vi "img test14(coutsegment attempt1).vi"() -> ()   [LabVIEW 2013]
uses:
  <vilib>/vision/NI_Vision_Development_Module.lvlib
panel:
  out "Waveform Chart":i32(graph)
  in  "ON":bool
  out "s? t:f 2":i32[](array[numeric])
  out "s? t:f":i32[](array[numeric])
  out "Top player court segment display":bool[][](array[boolean])
  out "Bottom player court segment display":bool[][](array[boolean])
  out "bottom player":cluster{"Numeric":dbl, "Numeric":dbl}[](array[cluster])
  out "top player":cluster{"Numeric":dbl, "Numeric":dbl}[](array[cluster])
  in  "playing":bool
  out "Top VIew":cluster{"Numeric":dbl, "Numeric":dbl}[](graph)
  out "Image 4":T1(plugin-control)
  in  "frame jump":i32=3
  in  "speed":u32(slide)=200
  in  "start":i32(slide) step=219843704 scale=0.0..42095.0
  out "Image 3":T1(plugin-control)
  in  "AVI Path":path=path "C:/Users/Kokum Weeratunga/Desktop/img processing/ChenJin vs HuYun.avi"
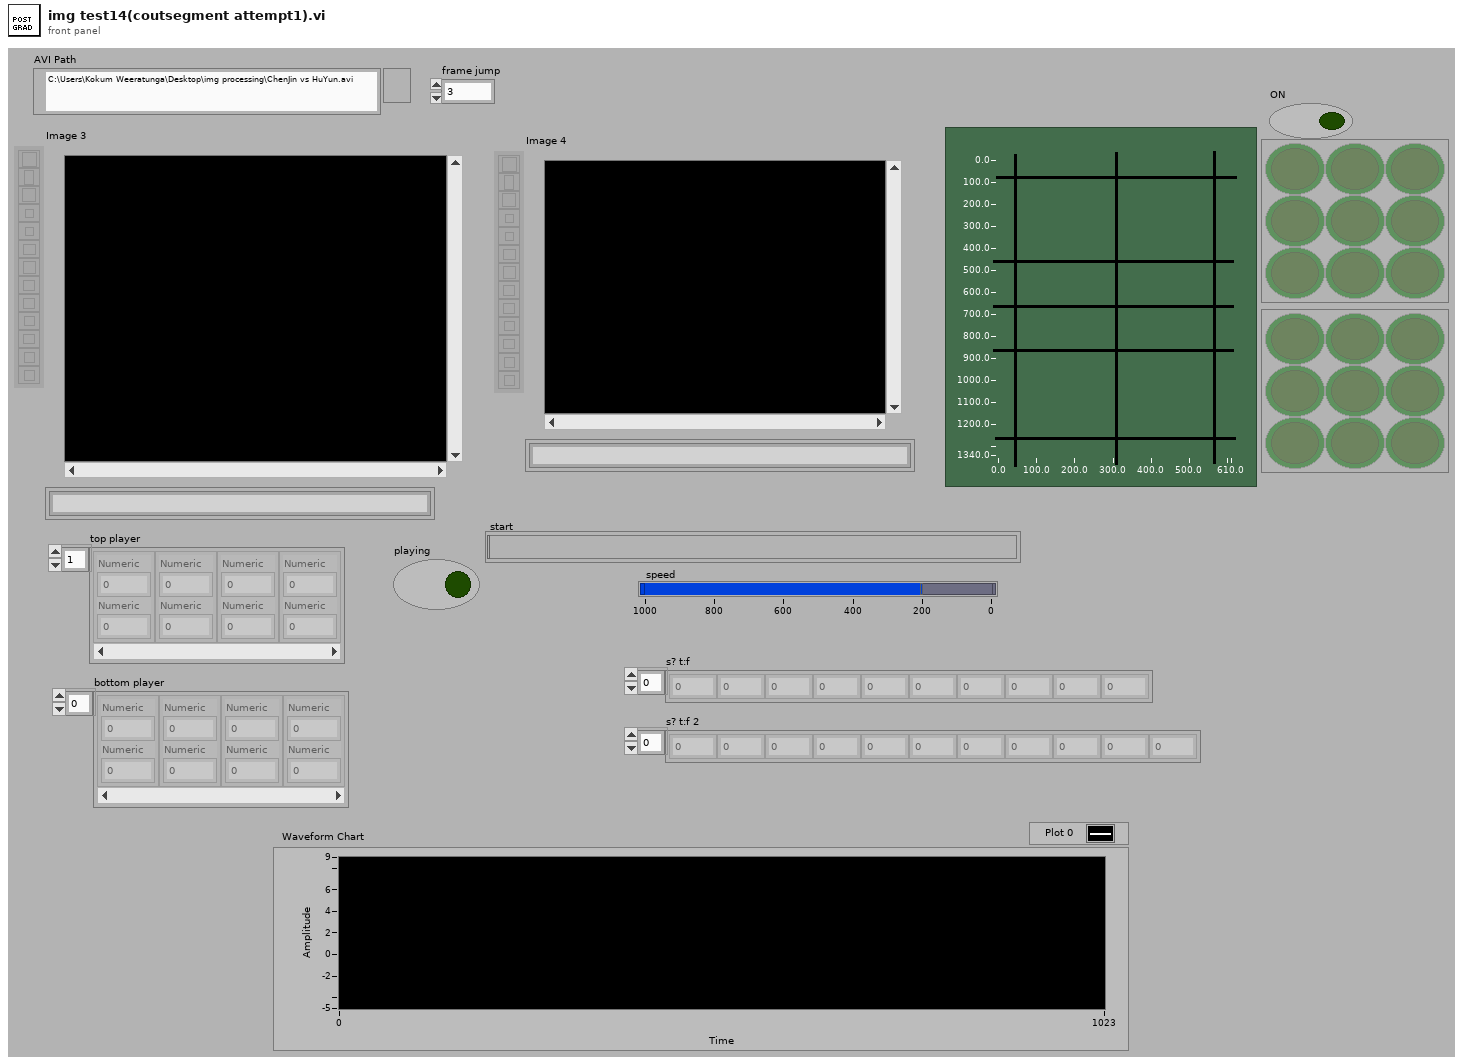
[diagram p1: front panel]
types:
  T1 = typedef "IMAQ Image.ctl" = refnum<image>
  T2 = typedef "Image Type" = u32
  T3 = typedef "AviRefnum.ctl" = refnum<k1>
  T4 = cluster{"width":u32, "height":u32, "framesPerSecond":u32, "compressionFilter":string, "hasData":bool}
  T5 = cluster{cluster{"X":sgl, "Y":sgl}[], cluster{i32, i32}[], "Unit":u32}
  T6 = cluster{"Origin Pixel":cluster{"X":sgl, "Y":sgl}, "Angle Relative to Horizontal (deg)":sgl, "Axis Reference":u32}
  T7 = typedef "Particle Parameters" = i32
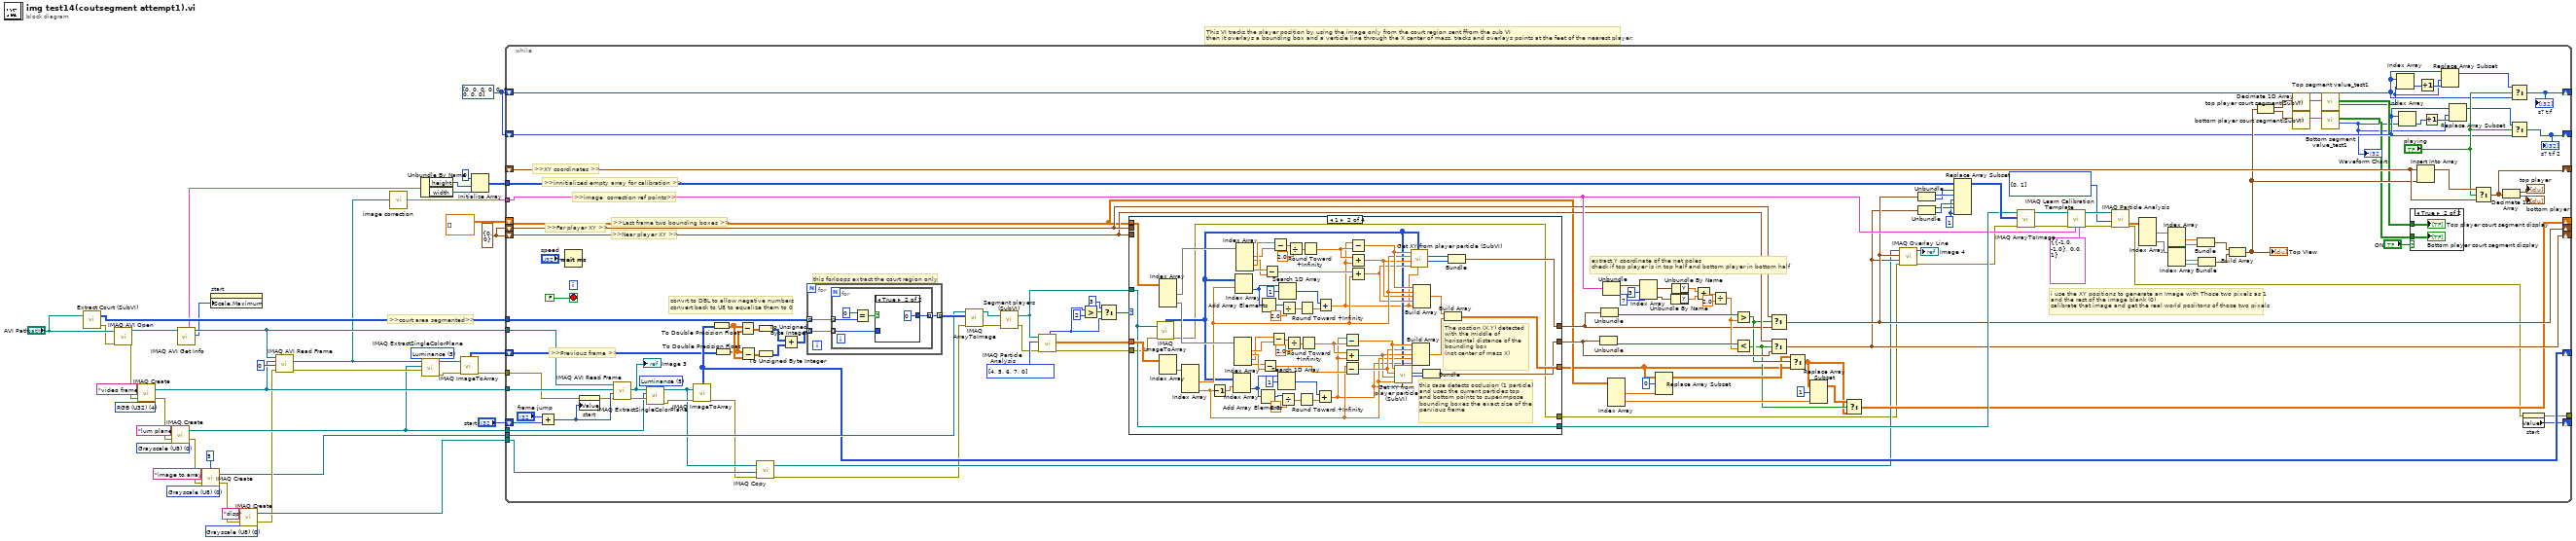
[diagram p0: block diagram]
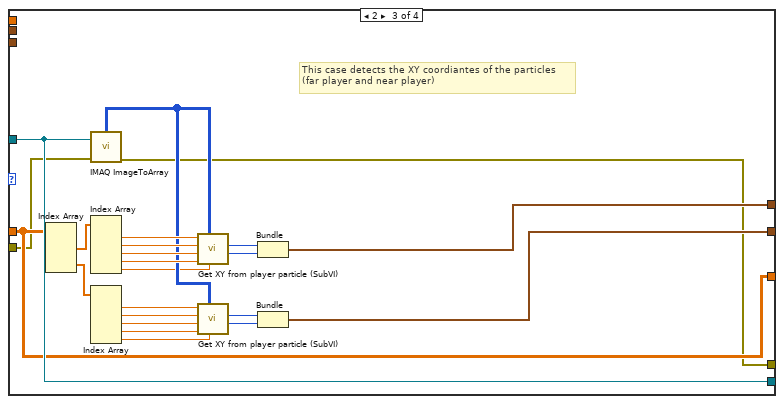
[diagram p4: hidden frame]
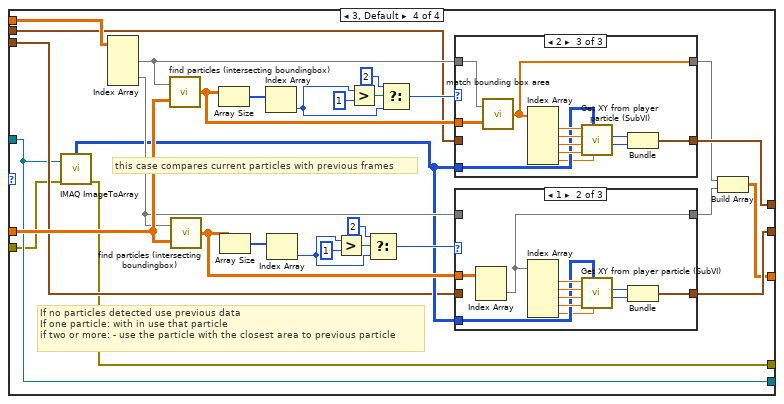
[diagram p5: hidden frame]
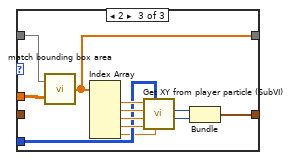
[diagram p7: hidden frame]
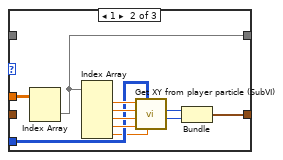
[diagram p9: hidden frame]
diagram:
  w1 = i32[] [0, 0, 0, 0, 0, 0, 0, 0, 0] ("input array")
  w14 = cluster{"X coordinate":i32, "Y coordinate":i32} {"X coordinate"=0, "Y coordinate"=0}
  w27 = T2 0 items=["Grayscale (U8)", "Grayscale (I16)", "Grayscale (SGL)", "Complex (CSG)", "RGB (U32)", "HSL (U32)", "RGB (U64)", "Grayscale (U16)"] ("Image Type")
  w34 = 5 items=["Red", "Green", "Blue", "Hue", "Saturation", "Luminance", "Value", "Intensity"] ("Color Plane")
  w35 = T2 0 items=["Grayscale (U8)", "Grayscale (I16)", "Grayscale (SGL)", "Complex (CSG)", "RGB (U32)", "HSL (U32)", "RGB (U64)", "Grayscale (U16)"] ("Image Type")
  w39 = T2 0 items=["Grayscale (U8)", "Grayscale (I16)", "Grayscale (SGL)", "Complex (CSG)", "RGB (U32)", "HSL (U32)", "RGB (U64)", "Grayscale (U16)"] ("Image Type")
  w37 = T2 4 items=["Grayscale (U8)", "Grayscale (I16)", "Grayscale (SGL)", "Complex (CSG)", "RGB (U32)", "HSL (U32)", "RGB (U64)", "Grayscale (U16)"] ("Image Type")
  # ">>court area segmented>>"
  # "This VI tracks the player position by using the image only from the court region sent ffrom the sub VI\nthen it overlays a bounding box and a verticle line through the X center of mass. tracks and overlays points at the feet of the nearest player."
  n1 = call "Extract Court (SubVI).vi"("AVI Path"="AVI Path") -> ("error out"=w41:errorcluster, "Court pixels out"=w17:u8[][])  [unwired: 1 in]
  n2 = call "IMAQ AVI Open"("error in (no error)"=w41, "AVI Path"="AVI Path") -> ("error out"=w23:errorcluster, "Avi Refnum"=w12:T3)  [unwired: 8 in]
  n3 = call "IMAQ Create"("Image Name"="video frame", "Image Type"=w37, "error in (no error)"=w23) -> ("New Image"=w31:T1, "error out"=w22:errorcluster)  [unwired: 2 in]
  n4 = call "IMAQ Create"("Image Name"="lum plane", "Image Type"=w39, "error in (no error)"=w22) -> ("New Image"=w30:T1, "error out"=w21:errorcluster)  [unwired: 2 in]
  n5 = call "IMAQ AVI Get Info"("Avi Refnum"=w12) -> ("Number of Frames"=w10:u32, "Avi Refnum (duplicate)"=w11:T3, "Frame Data"=w7:T4)  [unwired: 6 in, 2 out]
  n6 = call "IMAQ Create"("Border Size"=5, "Image Name"="image to array", "Image Type"=w35, "error in (no error)"=w21) -> ("New Image"=w16:T1, "error out"=w20:errorcluster)  [unwired: 1 in]
  n7 = property on="start" class="Slide (strict)"("Scale.Maximum"=w10) -> ()  [unwired: 2 in, 2 out]
  n8 = call "IMAQ Create"("Image Name"="disp", "Image Type"=w27, "error in (no error)"=w20) -> ("New Image"=w25:T1, "error out"=w19:errorcluster)  [unwired: 2 in]
  n9 = call "IMAQ AVI Read Frame"("error in (no error)"=w19, "Frame Number"=u32 0, "Image"=w31, "Avi Refnum"=w11) -> ("error out"=w33:errorcluster, "Image Out"=w3:T1)  [unwired: 4 in, 2 out]
  n10 = call "image correction.vi"("Image"=w3) -> ("ref points"=w2:T5)
  n11 = Unbundle By Name(w7) -> ("height"=w6:u32, "width"=w5:u32)
  n12 = call "IMAQ ExtractSingleColorPlane"("Color Plane"=w34, "error in (no error)"=w33, "Image Dst"=w30, "Image Src"=w3) -> ("error out"=w24:errorcluster, "Image Dst Out"=w28:T1)  [unwired: 6 in]
  n13 = call "IMAQ ImageToArray"("error in (no error)"=w24, "Image"=w28) -> ("error out"=w9:errorcluster, "Image Pixels (U8)"=w29:u8[][])  [unwired: 2 in, 3 out]
  n14 = Initialize Array(u8 0 ("element"), w6, w5) -> (w4:u8[][])
  n15 = while {
    tunnel: w11 -> [w134]
    tunnel: w31 -> [w153]
    tunnel: w17 -> [w169]
    tunnel: w30 -> [w154]
    tunnel: w16 -> [w166]
    shift-right: [w165] -> _
    shift-left: w29 -> [w164]
    tunnel: w25 -> [w137]
    shift-right: [w72] -> _
    shift-left: dbl[][] [] ("Particle Measurements (Pixels)") -> [w82]
    shift-right: [w86] -> _
    shift-left: w14 -> [w88]
    shift-right: [w84] -> _
    shift-left: w14 -> [w87]
    shift-right: [w130] -> _
    shift-left: "start" -> [w136]
    tunnel: w9 -> [w132]
    tunnel: w4 -> [w129]
    tunnel: w2 -> [w101]
    shift-right: [w104] -> _
    shift-left: _ -> [w107]
    shift-right: [w61] -> _
    shift-left: w1 -> [w52]
    shift-right: [w60] -> _
    shift-left: w1 -> [w56]
    tunnel: [w50] -> _
    stop <- FALSE stop-if-true
    w116 = T7[] [0, 1] items=["Center of Mass X", "Center of Mass Y", "First Pixel X", "First Pixel Y", "Bounding Rect Left", "Bounding Rect Top", "Bounding Rect Right", "Bounding Rect Bottom", "Max Feret Diameter Start X", "Max Feret Diameter Start Y", "Max Feret Diameter End X", "Max Feret Diameter End Y", "Max Horiz. Segment Length Left", "Max Horiz. Segment Length Right", "Max Horiz. Segment Length Row", "-", "Bounding Rect Width", "Bounding Rect Height", "Bounding Rect Diagonal", "Perimeter", "Convex Hull Perimeter", "Holes' Perimeter", "Max Feret Diameter", "Equivalent Ellipse Major Axis", "Equivalent Ellipse Minor Axis", "Equivalent Ellipse Minor Axis (Feret)", "Equivalent Rect Long Side", "Equivalent Rect Short Side", "Equivalent Rect Diagonal", "Equivalent Rect Short Side (Feret)", "Average Horiz. Segment Length", "Average Vert. Segment Length", "Hydraulic Radius", "Waddel Disk Diameter", "-", "Area", "Holes' Area", "Particle & Holes' Area", "Convex Hull Area", "Image Area", "-", "Number of Holes", "Number of Horiz. Segments", "Number of Vert. Segments", "-", "Orientation", "Max Feret Diameter Orientation", "-", "% Area/Image Area", "% Area/(Particle & Holes' Area)", "Ratio of Equivalent Ellipse Axes", "Ratio of Equivalent Rect Sides", "-", "Elongation Factor", "Compactness Factor", "Heywood Circularity Factor", "Type Factor", "-", "Sum X", "Sum Y", "Sum XX", "Sum XY", "Sum YY", "Sum XXX", "Sum XXY", "Sum XYY", "Sum YYY", "-", "Moment of Inertia XX", "Moment of Inertia XY", "Moment of Inertia YY", "Moment of Inertia XXX", "Moment of Inertia XXY", "Moment of Inertia XYY", "Moment of Inertia YYY", "Norm. Moment of Inertia XX", "Norm. Moment of Inertia XY", "Norm. Moment of Inertia YY", "Norm. Moment of Inertia XXX", "Norm. Moment of Inertia XXY", "Norm. Moment of Inertia XYY", "Norm. Moment of Inertia YYY", "Hu Moment 1", "Hu Moment 2", "Hu Moment 3", "Hu Moment 4", "Hu Moment 5", "Hu Moment 6", "Hu Moment 7"] ("Real-World Measurements")
    w124 = u8 1 ("new element/subarray")
    w155 = T7[] [4, 5, 6, 7, 0] items=["Center of Mass X", "Center of Mass Y", "First Pixel X", "First Pixel Y", "Bounding Rect Left", "Bounding Rect Top", "Bounding Rect Right", "Bounding Rect Bottom", "Max Feret Diameter Start X", "Max Feret Diameter Start Y", "Max Feret Diameter End X", "Max Feret Diameter End Y", "Max Horiz. Segment Length Left", "Max Horiz. Segment Length Right", "Max Horiz. Segment Length Row", "-", "Bounding Rect Width", "Bounding Rect Height", "Bounding Rect Diagonal", "Perimeter", "Convex Hull Perimeter", "Holes' Perimeter", "Max Feret Diameter", "Equivalent Ellipse Major Axis", "Equivalent Ellipse Minor Axis", "Equivalent Ellipse Minor Axis (Feret)", "Equivalent Rect Long Side", "Equivalent Rect Short Side", "Equivalent Rect Diagonal", "Equivalent Rect Short Side (Feret)", "Average Horiz. Segment Length", "Average Vert. Segment Length", "Hydraulic Radius", "Waddel Disk Diameter", "-", "Area", "Holes' Area", "Particle & Holes' Area", "Convex Hull Area", "Image Area", "-", "Number of Holes", "Number of Horiz. Segments", "Number of Vert. Segments", "-", "Orientation", "Max Feret Diameter Orientation", "-", "% Area/Image Area", "% Area/(Particle & Holes' Area)", "Ratio of Equivalent Ellipse Axes", "Ratio of Equivalent Rect Sides", "-", "Elongation Factor", "Compactness Factor", "Heywood Circularity Factor", "Type Factor", "-", "Sum X", "Sum Y", "Sum XX", "Sum XY", "Sum YY", "Sum XXX", "Sum XXY", "Sum XYY", "Sum YYY", "-", "Moment of Inertia XX", "Moment of Inertia XY", "Moment of Inertia YY", "Moment of Inertia XXX", "Moment of Inertia XXY", "Moment of Inertia XYY", "Moment of Inertia YYY", "Norm. Moment of Inertia XX", "Norm. Moment of Inertia XY", "Norm. Moment of Inertia YY", "Norm. Moment of Inertia XXX", "Norm. Moment of Inertia XXY", "Norm. Moment of Inertia XYY", "Norm. Moment of Inertia YYY", "Hu Moment 1", "Hu Moment 2", "Hu Moment 3", "Hu Moment 4", "Hu Moment 5", "Hu Moment 6", "Hu Moment 7"] ("Pixel Measurements")
    w170 = 5 items=["Red", "Green", "Blue", "Hue", "Saturation", "Luminance", "Value", "Intensity"] ("Color Plane")
    # ">>XY coordinates >>"
    # ">>innitialized empty array for calibration >>"
    # ">>image  correction ref points>>"
    # "extract Y coordinate of the net poles\ncheck if top player is in top half and bottom player in bottom half"
    # "i use the XY positions to generate an Image with Those two pixels as 1 \nand the rest of the image blank (0)\ncalibrate that image and get the real world posiitons of those two pixels"
    # ">>Last frame two bounding boxes >>"
    # ">>Far player XY >>"
    # ">>Near player XY >>"
    # ">>Previous frame >>"
    # "convrt to DBL to allow negative numbers\nconvert back to U8 to equalize them to 0"
    # "this forloops extract the court region only"
    n16 = Add(x="frame jump", y=w136) -> (x+y=w133:i32)
    n17 = Wait (ms)(milliseconds to wait="speed") -> ()  [unwired: 1 out]
    n18 = property on="start" class="Slide (strict)"(error in=w132, "Value"=w133) -> (error out=w131:errorcluster)  [unwired: 1 in, 1 out]
    n19 = call "IMAQ AVI Read Frame"("error in (no error)"=w131, "Frame Number"=w133, "Image"=w153, "Avi Refnum"=w134) -> ("error out"=w171:errorcluster, "Image Out"=w150:T1)  [unwired: 4 in, 2 out]
    "Image 3" <- w150
    n20 = call "IMAQ ExtractSingleColorPlane"("Color Plane"=w170, "error in (no error)"=w171, "Image Dst"=w154, "Image Src"=w150) -> ("error out"=w156:errorcluster, "Image Dst Out"=w138:T1)  [unwired: 6 in]
    n21 = call "IMAQ ImageToArray"("error in (no error)"=w156, "Image"=w138) -> ("error out"=w66:errorcluster, "Image Pixels (U8)"=w165:u8[][])  [unwired: 2 in, 3 out]
    n22 = To Double Precision Float(number=w165) -> (double precision float=w160:dbl[][])
    n23 = To Double Precision Float(number=w164) -> (double precision float=w159:dbl[][])
    n24 = Subtract(x=w160, y=w159) -> (x-y=w158:dbl[][])
    n25 = Subtract(x=w159, y=w160) -> (x-y=w157:dbl[][])
    n26 = call "IMAQ Copy"("error in (no error)"=w66, "Image Dst"=w137, "Image Src"=w138) -> ("error out"=w65:errorcluster, "Image Dst Out"=w67:T1)  [unwired: 3 in]
    n27 = To Unsigned Byte Integer(number=w158) -> (unsigned 8bit integer=w163:u8[][])
    n28 = To Unsigned Byte Integer(number=w157) -> (unsigned 8bit integer=w162:u8[][])
    n29 = Add(x=w163, y=w162) -> (x+y=w161:u8[][])
    n30 = for {
      tunnel: w169 -> [w344] mode=indexing
      tunnel: [w343] -> w167 mode=indexing
      tunnel: w161 -> [w342] mode=indexing
      n31 = for {
        tunnel: w344 -> [w349] mode=indexing
        tunnel: [w346] -> w343 mode=indexing
        tunnel: w342 -> [w345] mode=indexing
        n32 = Equal?(x=u8 0, y=w349) -> (x = y?=w347:bool)
        n33 = case shown="True" w347 {
          tunnel: [w350 u8 0 ("x")] -> w346
          tunnel: w345 -> [w350 _]
          frame False {
          }
          frame True {
          }
        }
      }
    }
    n34 = call "IMAQ ArrayToImage"("error in (no error)"=w65, "Image Pixels (U8)"=w167, "Image"=w166) -> ("error out"=w151:errorcluster, "Image Out"=w152:T1)  [unwired: 7 in]
    n35 = call "Segment players (SubVI).vi"("error In"=w151, "Image In"=w152) -> ("error out"=w144:errorcluster, "Image Out"=w142:T1)
    n36 = call "IMAQ Particle Analysis"("error in (no error)"=w144, "Pixel Measurements"=w155, "Image"=w142) -> ("error out"=w143:errorcluster, "Particle Measurements (Pixels)"=w141:dbl[][], "Number of Particles"=w146:i32)  [unwired: 3 in, 3 out]
    n37 = Greater?(x=w146, y=2) -> (0:w149:bool)
    n38 = Select(t=3 ("y"), s=w149, f=w146) -> (s? t:f=w145:i32)
    n39 = case shown="1" w145 {
      tunnel: [w177 w204 w258 w268] -> w122
      tunnel: w141 -> [_ w239 w244 w288]
      tunnel: w143 -> [w174 w180 w241 w264]
      tunnel: w142 -> [w177 w204 w258 w268]
      tunnel: [w175 w188 w246 w270] -> w83
      tunnel: [w176 w195 w245 w269] -> w85
      tunnel: [w178 w205 w244 w265] -> w71
      tunnel: w82 -> [w178 w229 _ w291]
      tunnel: w88 -> [w176 _ _ w276]
      tunnel: w87 -> [w175 _ _ w271]
      tunnel: [w174 w179 w240 w263] -> w63
      frame 0 {
        # "This case identifies frames where no particles are detected and keeps the same values from the\nprevious frame"
      }
      frame 1 {
        # "The postion (X,Y) detected with the middle of \nhorizontal distance of the bounding box\n(not center of mass X)"
        # "this case detects occlusion (1 particle)\nand uses the current particles top \nand bottom points to superimpose \nbounding boxes the exact size of the \npervious frame"
        n40 = call "IMAQ ImageToArray"("error in (no error)"=w180, "Image"=w204) -> ("error out"=w179:errorcluster, "Image Pixels (U8)"=w187:u8[][])  [unwired: 2 in, 3 out]
        n41 = Index Array(array=w229) -> (element #1=w237:dbl[], element #2=w209:dbl[])  [unwired: 4 in]
        n42 = Index Array(array=w239) -> (element=w238:dbl[])  [unwired: 2 in]
        n43 = Index Array(array=w238) -> (element #2=w200:dbl, element #4=w191:dbl)  [unwired: 4 in, 2 out]
        n44 = Decrement(x=w191) -> (x-1=w202:dbl)
        n45 = Index Array(array=w187, index (row)=w202) -> (element=w224:u8[])  [unwired: 1 in]
        n46 = Index Array(array=w209) -> (element #1=w213:dbl, element #2=w216:dbl, element #3=w212:dbl, element #4=w215:dbl)  [unwired: 4 in]
        n47 = Index Array(array=w187, index (row)=w200) -> (element=w217:u8[])  [unwired: 1 in]
        n48 = Index Array(array=w237) -> (element #1=w233:dbl, element #2=w230:dbl, element #3=w234:dbl, element #4=w231:dbl)  [unwired: 4 in]
        n49 = Add Array Elements(numeric array=w224) -> (sum=w225:u8)
        n50 = Add Array Elements(numeric array=w217) -> (sum=w221:u8)
        n51 = Subtract(x=w215, y=w216) -> (x-y=w203:dbl)
        n52 = Subtract(x=w231, y=w230) -> (x-y=w208:dbl)
        n53 = Subtract(x=w212, y=w213) -> (x-y=w211:dbl)
        n54 = Subtract(x=w234, y=w233) -> (x-y=w235:dbl)
        n55 = Search 1D Array(1D array=w224, element=u8 1) -> (index of element=w223:i32)  [unwired: 1 in]
        n56 = Search 1D Array(1D array=w217, element=u8 1) -> (index of element=w222:i32)  [unwired: 1 in]
        n57 = Divide(x=w225, y=2.0) -> (x/y=w226:dbl)
        n58 = Divide(x=w221, y=2.0) -> (x/y=w220:dbl)
        n59 = Divide(x=w211, y=2.0) -> (x/y=w214:dbl)
        n60 = Divide(x=w235, y=2.0) -> (x/y=w232:dbl)
        n61 = Round Toward +Infinity(x=w226) -> (ceil(x): smallest int >= x=w185:dbl)
        n62 = Round Toward +Infinity(x=w220) -> (ceil(x): smallest int >= x=w184:dbl)
        n63 = Round Toward +Infinity(x=w214) -> (ceil(x): smallest int >= x=w186:dbl)
        n64 = Round Toward +Infinity(x=w232) -> (ceil(x): smallest int >= x=w183:dbl)
        n65 = Add(x=w223, y=w185) -> (x+y=w181:dbl)
        n66 = Add(x=w222, y=w184) -> (x+y=w182:dbl)
        n67 = Subtract(x=w181, y=w186) -> (x-y=w194:dbl)
        n68 = Add(x=w186, y=w181) -> (x+y=w192:dbl)
        n69 = Subtract(x=w191, y=w203) -> (x-y=w193:dbl)
        n70 = Subtract(x=w182, y=w183) -> (x-y=w201:dbl)
        n71 = Add(x=w183, y=w182) -> (x+y=w199:dbl)
        n72 = Add(x=w208, y=w200) -> (x+y=w198:dbl)
        n73 = call "Get XY from player particle (SubVI).vi"("Center of mass X"=w181, "Image in Pixels (U8)"=w187, "Particle bounding rect bottom"=w191, "Particle bounding rect right"=w192, "Particle bounding rect top"=w193, "Particle bounding rect left"=w194) -> ("Y coordinate"=w189:i32, "X coordinate"=w190:i32)  [unwired: 2 in]
        n74 = call "Get XY from player particle (SubVI).vi"("Center of mass X"=w182, "Image in Pixels (U8)"=w187, "Particle bounding rect bottom"=w198, "Particle bounding rect right"=w199, "Particle bounding rect top"=w200, "Particle bounding rect left"=w201) -> ("Y coordinate"=w196:i32, "X coordinate"=w197:i32)  [unwired: 2 in]
        n75 = Build Array(w194, w193, w192, w191, w181) -> (w206:dbl[])
        n76 = Build Array(w201, w200, w199, w198, w182) -> (w207:dbl[])
        n77 = Bundle("X coordinate"=w190, "Y coordinate"=w189) -> (w188:cluster{"X coordinate":i32, "Y coordinate":i32})  [unwired: 1 in]
        n78 = Build Array(w207, w206) -> (w205:dbl[][])
        n79 = Bundle("X coordinate"=w197, "Y coordinate"=w196) -> (w195:cluster{"X coordinate":i32, "Y coordinate":i32})  [unwired: 1 in]
      }
      frame 2 {
        # "This case detects the XY coordiantes of the particles\n(far player and near player)"
        n80 = Index Array(array=w244) -> (element #1=w252:dbl[], element #2=w251:dbl[])  [unwired: 4 in]
        n81 = call "IMAQ ImageToArray"("error in (no error)"=w241, "Image"=w258) -> ("error out"=w240:errorcluster, "Image Pixels (U8)"=w253:u8[][])  [unwired: 2 in, 3 out]
        n82 = Index Array(array=w252) -> (element #1=w262:dbl, element #2=w261:dbl, element #3=w260:dbl, element #4=w259:dbl, element #5=w243:dbl)  [unwired: 5 in]
        n83 = Index Array(array=w251) -> (element #1=w254:dbl, element #2=w255:dbl, element #3=w256:dbl, element #4=w257:dbl, element #5=w242:dbl)  [unwired: 5 in]
        n84 = call "Get XY from player particle (SubVI).vi"("Center of mass X"=w243, "Image in Pixels (U8)"=w253, "Particle bounding rect bottom"=w259, "Particle bounding rect right"=w260, "Particle bounding rect top"=w261, "Particle bounding rect left"=w262) -> ("Y coordinate"=w249:i32, "X coordinate"=w250:i32)  [unwired: 2 in]
        n85 = call "Get XY from player particle (SubVI).vi"("Center of mass X"=w242, "Image in Pixels (U8)"=w253, "Particle bounding rect bottom"=w257, "Particle bounding rect right"=w256, "Particle bounding rect top"=w255, "Particle bounding rect left"=w254) -> ("Y coordinate"=w247:i32, "X coordinate"=w248:i32)  [unwired: 2 in]
        n86 = Bundle("X coordinate"=w250, "Y coordinate"=w249) -> (w245:cluster{"X coordinate":i32, "Y coordinate":i32})  [unwired: 1 in]
        n87 = Bundle("X coordinate"=w248, "Y coordinate"=w247) -> (w246:cluster{"X coordinate":i32, "Y coordinate":i32})  [unwired: 1 in]
      }
      frame 3, Default {
        # "If no particles detected use previous data\nIf one particle: with in use that particle\nif two or more: - use the particle with the closest area to previous particle"
        # "this case compares current particles with previous frames"
        n88 = call "IMAQ ImageToArray"("error in (no error)"=w264, "Image"=w268) -> ("error out"=w263:errorcluster, "Image Pixels (U8)"=w272:u8[][])  [unwired: 2 in, 3 out]
        n89 = Index Array(array=w291) -> (element #1=w287:dbl[], element #2=w275:dbl[])  [unwired: 4 in]
        n90 = call "find particles (intersecting boundingbox).vi"("Particle Measurements in (bounding boxes)"=w288, "bounding box in"=w287) -> ("Particles within bounding box"=w286:dbl[][])
        n91 = call "find particles (intersecting boundingbox).vi"("Particle Measurements in (bounding boxes)"=w288, "bounding box in"=w275) -> ("Particles within bounding box"=w273:dbl[][])
        n92 = Array Size(array=w286) -> (size(s)=w290:i32[])
        n93 = Array Size(array=w273) -> (size(s)=w289:i32[])
        n94 = Index Array(array=w290) -> (element=w278:i32)  [unwired: 1 in]
        n95 = Index Array(array=w289) -> (element=w279:i32)  [unwired: 1 in]
        n96 = Greater?(x=w279, y=1) -> (0:w282:bool)
        n97 = Greater?(x=w278, y=1) -> (0:w283:bool)
        n98 = Select(t=2 ("y"), s=w282, f=w279) -> (s? t:f=w274:i32)
        n99 = Select(t=2 ("y"), s=w283, f=w278) -> (s? t:f=w277:i32)
        n100 = case shown="2" w277 {
          tunnel: w287 -> [w318 _ w333]
          tunnel: w286 -> [_ w329 w332]
          tunnel: [w318 w320 w331] -> w267
          tunnel: w272 -> [_ w322 w335]
          tunnel: [w317 w321 w334] -> w269
          tunnel: w276 -> [w317 _ _]
          frame 0, Default {
          }
          frame 1 {
            n101 = Index Array(array=w329) -> (element=w320:dbl[])  [unwired: 2 in]
            n102 = Index Array(array=w320) -> (element #1=w326:dbl, element #2=w325:dbl, element #3=w324:dbl, element #4=w323:dbl, element #5=w319:dbl)  [unwired: 5 in]
            n103 = call "Get XY from player particle (SubVI).vi"("Center of mass X"=w319, "Image in Pixels (U8)"=w322, "Particle bounding rect bottom"=w323, "Particle bounding rect right"=w324, "Particle bounding rect top"=w325, "Particle bounding rect left"=w326) -> ("Y coordinate"=w327:i32, "X coordinate"=w328:i32)  [unwired: 2 in]
            n104 = Bundle("X coordinate"=w328, "Y coordinate"=w327) -> (w321:cluster{"X coordinate":i32, "Y coordinate":i32})  [unwired: 1 in]
          }
          frame 2 {
            n105 = call "match bounding box area.vi"("particle measurements (bounding box)"=w332, "bounding box in"=w333) -> ("matching bounding box"=w331:dbl[])
            n106 = Index Array(array=w331) -> (element #1=w339:dbl, element #2=w338:dbl, element #3=w337:dbl, element #4=w336:dbl, element #5=w330:dbl)  [unwired: 5 in]
            n107 = call "Get XY from player particle (SubVI).vi"("Center of mass X"=w330, "Image in Pixels (U8)"=w335, "Particle bounding rect bottom"=w336, "Particle bounding rect right"=w337, "Particle bounding rect top"=w338, "Particle bounding rect left"=w339) -> ("Y coordinate"=w340:i32, "X coordinate"=w341:i32)  [unwired: 2 in]
            n108 = Bundle("X coordinate"=w341, "Y coordinate"=w340) -> (w334:cluster{"X coordinate":i32, "Y coordinate":i32})  [unwired: 1 in]
          }
        }
        n109 = case shown="1" w274 {
          tunnel: w275 -> [w293 _ w308]
          tunnel: w273 -> [_ w304 w307]
          tunnel: [w293 w295 w306] -> w266
          tunnel: w272 -> [_ w297 w310]
          tunnel: [w292 w296 w309] -> w270
          tunnel: w271 -> [w292 _ _]
          frame 0, Default {
          }
          frame 1 {
            n110 = Index Array(array=w304) -> (element=w295:dbl[])  [unwired: 2 in]
            n111 = Index Array(array=w295) -> (element #1=w301:dbl, element #2=w300:dbl, element #3=w299:dbl, element #4=w298:dbl, element #5=w294:dbl)  [unwired: 5 in]
            n112 = call "Get XY from player particle (SubVI).vi"("Center of mass X"=w294, "Image in Pixels (U8)"=w297, "Particle bounding rect bottom"=w298, "Particle bounding rect right"=w299, "Particle bounding rect top"=w300, "Particle bounding rect left"=w301) -> ("Y coordinate"=w302:i32, "X coordinate"=w303:i32)  [unwired: 2 in]
            n113 = Bundle("X coordinate"=w303, "Y coordinate"=w302) -> (w296:cluster{"X coordinate":i32, "Y coordinate":i32})  [unwired: 1 in]
          }
          frame 2 {
            n114 = call "match bounding box area.vi"("particle measurements (bounding box)"=w307, "bounding box in"=w308) -> ("matching bounding box"=w306:dbl[])
            n115 = Index Array(array=w306) -> (element #1=w314:dbl, element #2=w313:dbl, element #3=w312:dbl, element #4=w311:dbl, element #5=w305:dbl)  [unwired: 5 in]
            n116 = call "Get XY from player particle (SubVI).vi"("Center of mass X"=w305, "Image in Pixels (U8)"=w310, "Particle bounding rect bottom"=w311, "Particle bounding rect right"=w312, "Particle bounding rect top"=w313, "Particle bounding rect left"=w314) -> ("Y coordinate"=w315:i32, "X coordinate"=w316:i32)  [unwired: 2 in]
            n117 = Bundle("X coordinate"=w316, "Y coordinate"=w315) -> (w309:cluster{"X coordinate":i32, "Y coordinate":i32})  [unwired: 1 in]
          }
        }
        n118 = Build Array(w267, w266) -> (w265:dbl[][])
      }
    }
    n119 = Unbundle(w83) -> ("Y coordinate"=w90:i32)  [unwired: 1 out]
    n120 = Unbundle(w85) -> ("Y coordinate"=w91:i32)  [unwired: 1 out]
    n121 = Unbundle(w101) -> (w100:cluster{"X":sgl, "Y":sgl}[])  [unwired: 2 out]
    n122 = Index Array(array=w82) -> (element #1=w80:dbl[], element #2=w76:dbl[])  [unwired: 4 in]
    n123 = Index Array(array=w100, index #1=3 ("index"), index #2=7 ("index")) -> (element #1=w97:cluster{"X":sgl, "Y":sgl}, element #2=w96:cluster{"X":sgl, "Y":sgl})
    n124 = Replace Array Subset(array=w71, new element=w80, index (row)=0) -> (w79:dbl[][])  [unwired: 1 in]
    n125 = Unbundle By Name(w96) -> ("Y"=w94:sgl)
    n126 = Unbundle By Name(w97) -> ("Y"=w95:sgl)
    n127 = Add(x=w95, y=w94) -> (x+y=w93:sgl)
    n128 = Divide(x=w93, y=sgl 2.0) -> (x/y=w89:sgl)
    n129 = Greater?(x=w91, y=w89) -> (0:w81:bool)
    n130 = Less?(x=w90, y=w89) -> (x < y?=w74:bool)
    n131 = Select(t=w88, s=w81, f=w85) -> (s? t:f=w86:cluster{"X coordinate":i32, "Y coordinate":i32})
    n132 = Select(t=w87, s=w74, f=w83) -> (s? t:f=w84:cluster{"X coordinate":i32, "Y coordinate":i32})
    n133 = Select(t=w79, s=w81, f=w71) -> (s? t:f=w73:dbl[][])
    n134 = Replace Array Subset(array=w73, new element=w76, index (row)=1) -> (w75:dbl[][])  [unwired: 1 in]
    n135 = Select(t=w75, s=w74, f=w73) -> (s? t:f=w72:dbl[][])
    n136 = call "IMAQ Overlay Line"("error in (no error)"=w63, "End Point"=w84, "Start Point"=w86, "Image"=w67) -> ("error out"=w64:errorcluster, "Image Out"=→"Image 4":T1)  [unwired: 6 in]
    n137 = Unbundle(w84) -> ("X coordinate"=w125:i32, "Y coordinate"=w126:i32)
    n138 = Unbundle(w86) -> ("X coordinate"=w128:i32, "Y coordinate"=w127:i32)
    n139 = Replace Array Subset(array=w129, new element #1=w124, index (row) #1=w127, index (col) #1=w128, new element #2=w124, index (row) #2=w126, index (col) #2=w125) -> (w123:u8[][])
    n140 = call "IMAQ ArrayToImage"("error in (no error)"=w64, "Image Pixels (U8)"=w123, "Image"=w122) -> ("error out"=w119:errorcluster, "Image Out"=w120:T1)  [unwired: 7 in]
    n141 = call "IMAQ Learn Calibration Template"("Calibration Axis Info"=T6 {"Origin Pixel"={"X"=-1.0, "Y"=-1.0}, "Angle Relative to Horizontal (deg)"=0.0, "Axis Reference"=1}, "Reference Points"=w101, "error in (no error)"=w119, "Image"=w120) -> ("error out"=w118:errorcluster, "Calibrated Image"=w117:T1)  [unwired: 5 in, 1 out]
    n142 = call "IMAQ Particle Analysis"("error in (no error)"=w118, "Real-World Measurements"=w116, "Image"=w117) -> ("error out"=w51:errorcluster, "Particle Measurements (Real-World)"=w115:dbl[][])  [unwired: 3 in, 4 out]
    n143 = Index Array(array=w115) -> (element #1=w114:dbl[], element #2=w113:dbl[])  [unwired: 4 in]
    n144 = Index Array(array=w114) -> (element #1=w110:dbl, element #2=w109:dbl)  [unwired: 2 in]
    n145 = Index Array(array=w113) -> (element #1=w111:dbl, element #2=w112:dbl)  [unwired: 2 in]
    n146 = Bundle("Numeric"=w110, "Numeric"=w109) -> (w106:cluster{"Numeric":dbl, "Numeric":dbl})  [unwired: 1 in]
    n147 = Bundle("Numeric"=w111, "Numeric"=w112) -> (w105:cluster{"Numeric":dbl, "Numeric":dbl})  [unwired: 1 in]
    n148 = Build Array(w106, w105) -> (w70:cluster{"Numeric":dbl, "Numeric":dbl}[])
    "Top VIew" <- w70
    n149 = Decimate 1D Array(w70) -> (w68:cluster{"Numeric":dbl, "Numeric":dbl}[], w69:cluster{"Numeric":dbl, "Numeric":dbl}[])
    n150 = call "top player court segment(SubVI).vi"("Top player position"=w68) -> ("Top player segment position"=w48:string)  [unwired: 10 in]
    n151 = call "bottom player court segment(SubVI).vi"("Bottom player position"=w69) -> ("Bottom player segment position"=w45:string)  [unwired: 10 in]
    n152 = call "Top segment value_test1.vi"("Top player segment position"=w48) -> ("Top player segment value"=w46:i32, "Top player court segment display"=w47:bool[][])  [unwired: 9 in]
    n153 = call "Bottom segment value_test1.vi"("Bottom player segment position"=w45) -> ("Bottom player segment"=w43:i32, "Bottom player court segment display"=w44:bool[][])  [unwired: 9 in]
    "Waveform Chart" <- w43
    n154 = Index Array(array=w56, index=w46) -> (element=w58:i32)
    n155 = Index Array(array=w52, index=w43) -> (element=w55:i32)
    n156 = case shown="True" "ON" {
      tunnel: w47 -> [_ w173]
      tunnel: w44 -> [_ w172]
      frame False {
      }
      frame True {
        "Bottom player court segment display" <- w172
        "Top player court segment display" <- w173
      }
    }
    n157 = Insert Into Array(array=w107, new element=w70) -> (w108:cluster{"Numeric":dbl, "Numeric":dbl}[])  [unwired: 1 in]
    n158 = Increment(x=w58) -> (x+1=w59:i32)
    n159 = Increment(x=w55) -> (x+1=w54:i32)
    n160 = Replace Array Subset(array=w56, new element=w59, index=w46) -> (w57:i32[])
    n161 = Replace Array Subset(array=w52, new element=w54, index=w43) -> (w53:i32[])
    n162 = Select(t=w108, s="playing", f=w107) -> (s? t:f=w104:cluster{"Numeric":dbl, "Numeric":dbl}[])
    n163 = Decimate 1D Array(w104) -> (→"top player":cluster{"Numeric":dbl, "Numeric":dbl}[], →"bottom player":cluster{"Numeric":dbl, "Numeric":dbl}[])
    n164 = Select(t=w57, s="playing", f=w56) -> (s? t:f=w60:i32[])
    "s? t:f" <- w60
    n165 = Select(t=w53, s="playing", f=w52) -> (s? t:f=w61:i32[])
    "s? t:f 2" <- w61
    n166 = property on="start" class="Slide (strict)"(error in=w51) -> (error out=w50:errorcluster, "Value"=w130:i32)  [unwired: 1 in, 1 out]
  }
